vi "V-Meter Adjust Measure1.vi"(8 "error in (no error)":errorcluster, 11 "VISA resource name in":refnum<visa-resource-name>) -> (0 "error out":errorcluster, 3 "VISA resource name out":refnum<visa-resource-name>)   [LabVIEW 2016, in "Hall Effect Library.lvlib"]
uses:
  Hall Effect Library.lvlib
  Global Variables/Instruments.vi
  Global Variables/Test Settings.vi
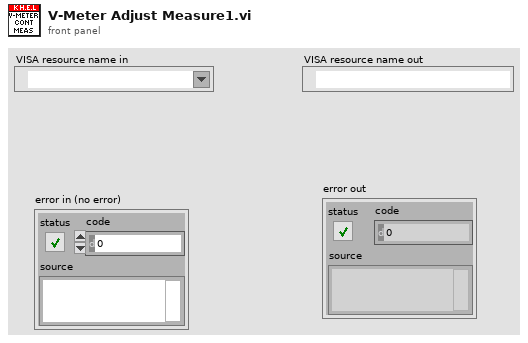
[diagram p1: front panel]
types:
  T1 = typedef "Hall Effect Library.lvlib/Voltmeters.ctl" = enum16{"2000", "2182A", "3706A"}
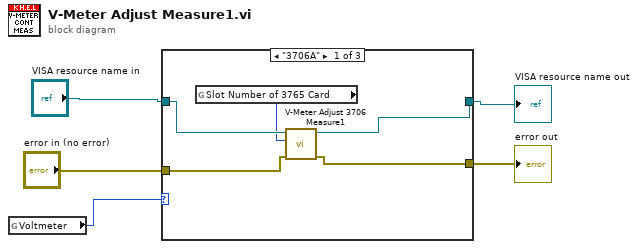
[diagram p0: block diagram]
diagram:
  n1 = global read "Instruments.vi" "Voltmeter"() -> (w3:T1)
  n2 = case shown="\"3706A\"" w3 {
    tunnel: "VISA resource name in" -> [w10 w12 w14]
    tunnel: "error in (no error)" -> [w9 w11 w13]
    tunnel: [w8 w12 w14] -> w2
    tunnel: [w7 w11 w13] -> w1
    frame "3706A" {
      n3 = global read "Test Settings.vi" "Slot Number of 3765 Card"() -> (w6:u32)
      n4 = call "V-Meter Adjust 3706 Measure1.vi"("error in (no error)"=w9, "Slot Number"=w6, "VISA resource name in"=w10) -> ("error out"=w7:errorcluster, "VISA resource name out"=w8:refnum<visa-resource-name>)  [unwired: 7 in]
    }
    frame "2000", Default {
    }
    frame "2182A" {
    }
  }
  "error out" <- w1
  "VISA resource name out" <- w2
